vi "ProgramState.vi"(0 "Universal Robot.lvclass in":refnum<class "Universal Robot.lvclass">, 5 "error in (no error)":errorcluster) -> (14 "Universal Robot.lvclass out":refnum<class "Universal Robot.lvclass">, 16 "programState out":T1, 19 "error out":errorcluster)   [LabVIEW 2019, in "Universal Robot.lvclass"]
uses:
  Universal Robot.lvclass
  ProgramState.ctl
  Universal Robot.lvclass/Universal Robot.ctl
  Client Interfaces/Dashboard Server/Dashboard Server.lvclass
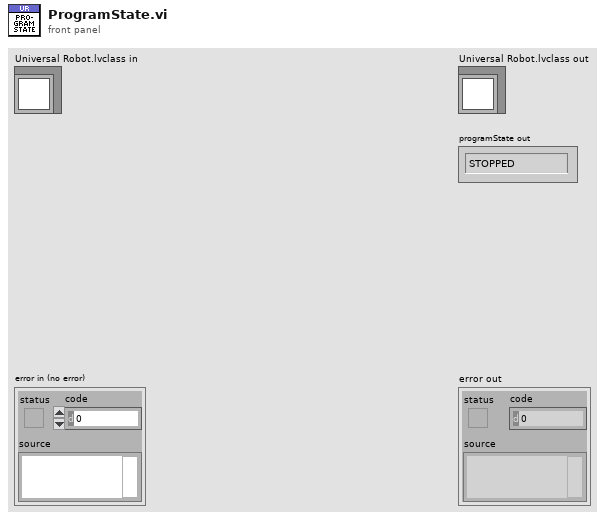
[diagram p1: front panel]
types:
  T1 = typedef "Universal Robot.lvclass/ProgramState.ctl" = enum16{"STOPPED", "PLAYING", "PAUSE"}
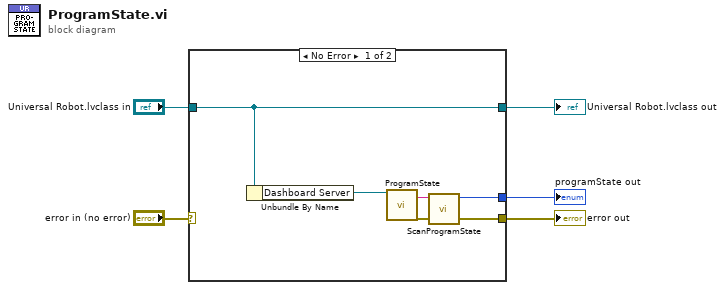
[diagram p0: block diagram]
diagram:
  n1 = case shown="No Error" "error in (no error)" {
    selector: "error in (no error)" -> [_ w12]
    tunnel: [w7 w12] -> w4
    tunnel: "Universal Robot.lvclass in" -> [w10 w11]
    tunnel: [w10 w11] -> w2
    tunnel: [w6 _] -> w1
    frame No Error {
      n2 = Unbundle By Name(w10) -> ("Dashboard Server"=w8:refnum<class "Dashboard Server.lvclass">)
      n3 = call-dynamic "ProgramState.vi"("DashboardServer in"=w8) -> ("programState"=w9:string, "error out"=w7:errorcluster)  [unwired: 16 in, 1 out]
      n4 = call "ScanProgramState.vi"("programState in"=w9) -> ("programState out"=w6:T1)  [unwired: 10 in]
    }
    frame Error {
    }
  }
  "error out" <- w4
  "Universal Robot.lvclass out" <- w2
  "programState out" <- w1
